vi "Vision Research Phantom Series PhSetCameraTime.vi"(0 "CN in":u32=1, 5 "Error In (no error)":errorcluster) -> (14 "CN out":u32=1, 19 "Error Out":errorcluster)   [LabVIEW 2013, in "VRI.lvlib"]
doc: "PhCon.dll\n\nPhSetCameraTime\nHRESULT PhSetCameraTime(UINT CN, time_t Time);\n\nParameters Description\nCN (in) Camera number.\nTime (in) Seconds from Jan 1 1970 0:0:0.\nReturn HRESULT (0=Ok)\nComments Set the camera clock (for example from the computer clock).\n This cannot be done when the IRIG signal is present.\n To avoid IRIG and nonIRIG time discordance and to meet\n the customers expectations the time displayed in the\n Phantom software and on the video monitor is the local time.\n\nWritten by:\nBLOOMY CONTROLS, INC\nWINDSOR, CT 06095, USA\n860-298-9925\nwww.bloomy.com\nV1.0.0\nMay, 2004"
uses:
  VRI.lvlib
  Phantom DLLs/PhCon.dll
panel:
  in  "Time":i32
  out "Time out":i32
  # "For instructions on the use of this VI, press Ctrl+H to display the help window and move the mouse over the icon, controls, and indicators"
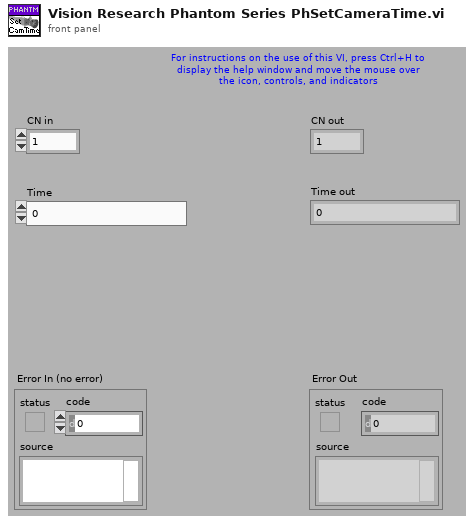
[diagram p1: front panel]
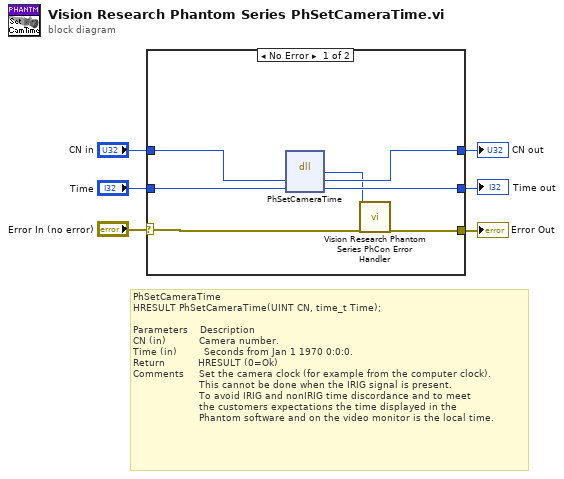
[diagram p0: block diagram]
diagram:
  # "PhSetCameraTime\nHRESULT PhSetCameraTime(UINT CN, time_t Time);\n\nParameters    Description\nCN (in)           Camera number.\nTime (in)         Seconds from Jan 1 1970 0:0:0.\nReturn           HRESULT (0=Ok)\nComments     Set the camera clock (for example from the computer clock).\n                      This cannot be done when the IRIG signal is present.\n                      To avoid IRIG and nonIRIG time discordance and to meet\n                      the customers expectations the time displayed in the\n                      Phantom software and on the video monitor is the local time."
  n1 = case shown="No Error" "Error In (no error)" {
    selector: "Error In (no error)" -> [w13 w16]
    tunnel: [w12 w16] -> w5
    tunnel: "CN in" -> [w11 w15]
    tunnel: [w10 w15] -> w3
    tunnel: [w9 w14] -> w2
    tunnel: "Time" -> [w8 w14]
    frame No Error {
      n2 = dll-call lib="C:/Projects/SDK/32-bit/Vision Research Phantom Series Labview Driver/Phantom DLLs/PhCon.dll" fn="PhSetCameraTime"("CN"=w11, "Time"=w8) -> ("HRESULT"=w7:i32, "CN"=w10:u32, "Time"=w9:i32)  [unwired: 3 in, 2 out]
      n3 = call "Vision Research Phantom Series PhCon Error Handler.vi"("ErrNo"=w7, "Error In (no error)"=w13) -> ("Error Out"=w12:errorcluster)  [unwired: 17 out]
    }
    frame Error {
    }
  }
  "Error Out" <- w5
  "CN out" <- w3
  "Time out" <- w2
